vi "WhileLoop-Demo1.vi"() -> ()   [LabVIEW 2018]
panel:
  in  "stop":bool
  out "Loop Count":dbl
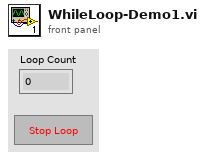
[diagram p1: front panel]
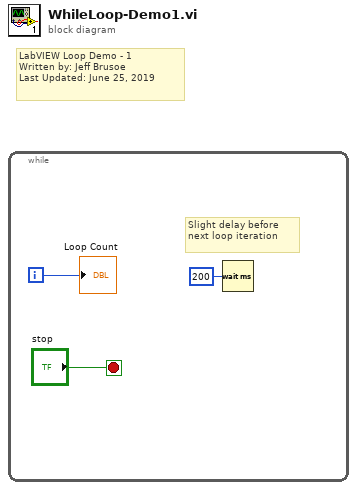
[diagram p0: block diagram]
diagram:
  # "LabVIEW Loop Demo - 1\nWritten by: Jeff Brusoe\nLast Updated: June 25, 2019"
  n1 = while {
    i -> [w3]
    stop <- "stop" stop-if-true
    # "Slight delay before\nnext loop iteration"
    n2 = Wait (ms)(milliseconds to wait=u32 200) -> ()  [unwired: 1 out]
    "Loop Count" <- w3
  }
